vi "convertXMLStringToTimestamp.vi"(7 "dataType":timestamp, 8 "error in (no error)":errorcluster, 10 "XMLContents In":string) -> (0 "error out":errorcluster, 2 "Timestamp Out":timestamp)   [LabVIEW 2012, in "XMLStringToDataConverter.lvlib"]
uses:
  <userlib>/Common/XML/XMLStringToDataConverter/XMLStringToDataConverter.lvlib
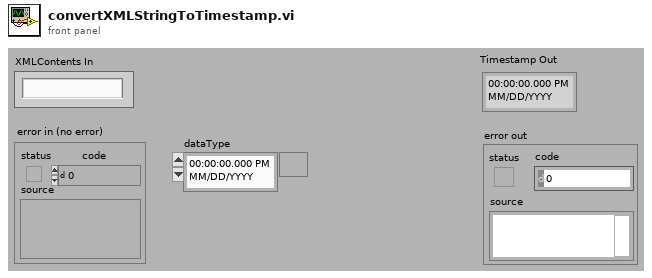
[diagram p1: front panel]
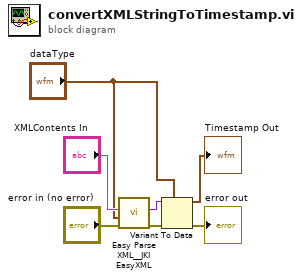
[diagram p0: block diagram]
diagram:
  n1 = call <vilib>:"Easy Parse XML__JKI EasyXML.vi"("error in (no error)"="error in (no error)", "LabVIEW Data (Type)"="dataType", "XML String"="XMLContents In") -> ("error out"=w5:errorcluster, "LabVIEW Data"=w3:variant)  [unwired: 7 in]
  n2 = Variant To Data(error in=w5, type="dataType", Variant=w3) -> (data=→"Timestamp Out":timestamp, error out=→"error out":errorcluster)
